vi "Log Error.vi"(8 "error in (no error)":errorcluster, 9 "Error Data":T1, 10 "file path (use dialog)":path, 11 "ATM Controller in":refnum<class "ATM Controller.lvclass">) -> (0 "error out":errorcluster, 3 "ATM Controller out":refnum<class "ATM Controller.lvclass">)   [LabVIEW 2019, in "ATM Controller.lvlib" / "ATM Controller.lvclass"]
uses:
  ATM Controller.lvclass
  Error Data.ctl
  Error Level.ctl
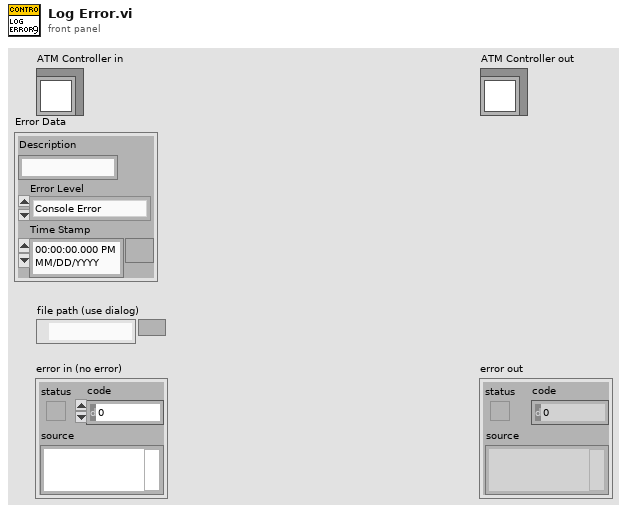
[diagram p1: front panel]
types:
  T1 = typedef "ATM Controller.lvlib/ATM Controller.lvclass/Error Data.ctl" = cluster{"Description":string, "Error Level":T2, "Time Stamp":timestamp}
  T2 = typedef "ATM Controller.lvlib/ATM Controller.lvclass/Error Level.ctl" = enum16{"Console Error", "Sensor Interface Error", "Process Step Error"}
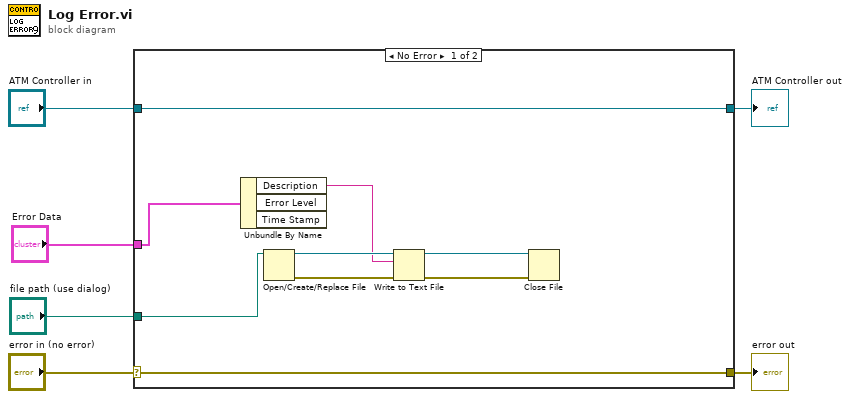
[diagram p0: block diagram]
diagram:
  n1 = case shown="No Error" "error in (no error)" {
    selector: "error in (no error)" -> [w14 w17]
    tunnel: [w14 w17] -> w5
    tunnel: [w15 w16] -> w3
    tunnel: "ATM Controller in" -> [w15 w16]
    tunnel: "Error Data" -> [w8 _]
    tunnel: "file path (use dialog)" -> [w9 _]
    frame No Error {
      n2 = Unbundle By Name(w8) -> ("Description"=w7:string)  [unwired: 2 out]
      n3 = Open/Create/Replace File(file path (use dialog)=w9) -> (refnum out=w13:refnum<file>, error out=w11:errorcluster)  [unwired: 5 in, 1 out]
      n4 = Write to Text File(file (use dialog)=w13, text=w7, error in=w11) -> (refnum out=w12:refnum<file>, error out=w10:errorcluster)  [unwired: 1 in, 1 out]
      n5 = Close File(refnum=w12, error in=w10) -> ()  [unwired: 2 out]
    }
    frame Error {
    }
  }
  "error out" <- w5
  "ATM Controller out" <- w3
